vi "OP600ZP_CLUSTER_ISO.vi"(5 "Tableau 3":string[][](array[string]), 10 "Numérique en entrée":i32, 11 "MESURES ISO":cluster{string, string, string, string}) -> (1 "Chaîne":string, 2 "Tableau 2":string[][](array[string]), 3 "Numérique en sortie":i32, 4 "Tableau":bool[](array[boolean]))   [LabVIEW 2020]
uses:
  VG/PackType.vi
  OP500/SubVI/OP500ZP_VGConf.vi
  OP600ZP_VGConf.vi
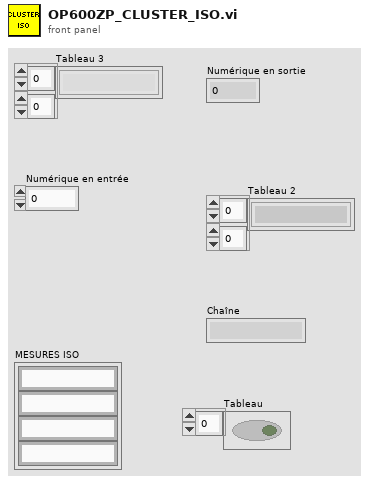
[diagram p1: front panel]
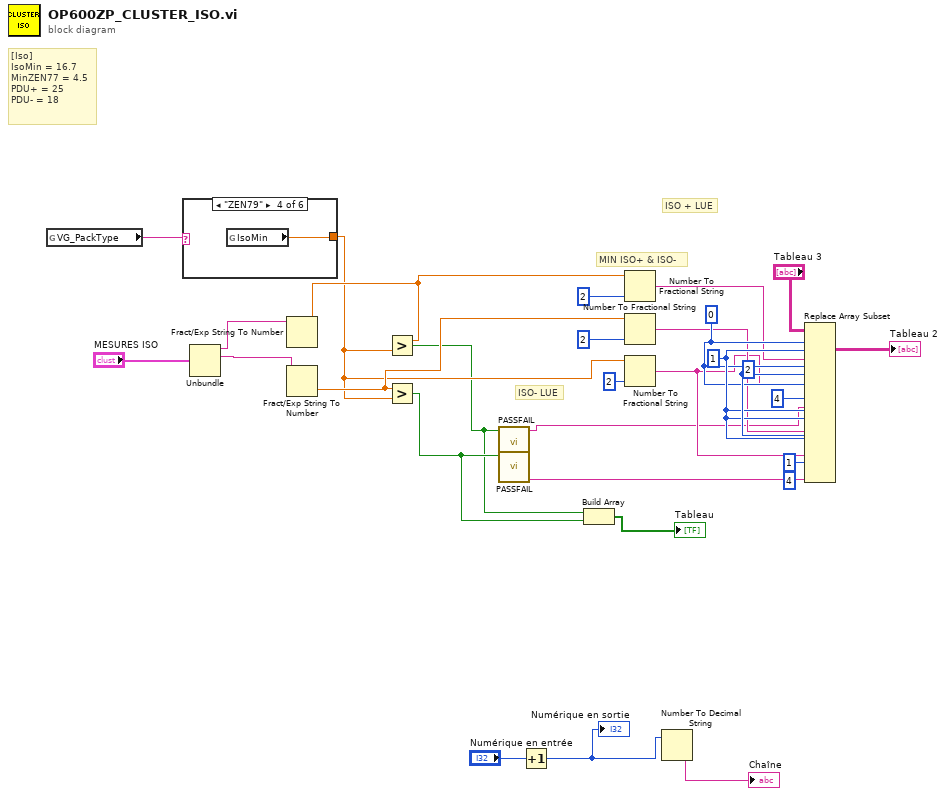
[diagram p0: block diagram]
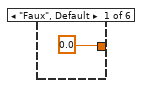
[diagram p2: hidden frame]
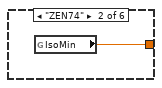
[diagram p3: hidden frame]
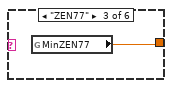
[diagram p4: hidden frame]
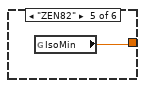
[diagram p5: hidden frame]
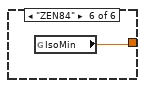
[diagram p6: hidden frame]
diagram:
  w29 = 2 ("disabled index (col)")
  w28 = 1 ("disabled index (col)")
  w26 = 0 ("index (row)")
  # "[Iso]\nIsoMin = 16.7\nMinZEN77 = 4.5\nPDU+ = 25\nPDU- = 18"
  # "ISO- LUE"
  # "ISO + LUE"
  # "MIN ISO+ & ISO-"
  n1 = global read "PackType.vi" "VG_PackType"() -> (w17:string)
  n2 = case shown="\"ZEN79\"" w17 {
    tunnel: [0.0 ("IsoMin") w31 w32 w33 w34 w35] -> w10
    frame "Faux", Default {
    }
    frame "ZEN74" {
      n3 = global read "OP500ZP_VGConf.vi" "IsoMin"() -> (w31:dbl)
    }
    frame "ZEN77" {
      n4 = global read "OP600ZP_VGConf.vi" "MinZEN77"() -> (w32:dbl)
    }
    frame "ZEN79" {
      n5 = global read "OP600ZP_VGConf.vi" "IsoMin"() -> (w33:dbl)
    }
    frame "ZEN82" {
      n6 = global read "OP500ZP_VGConf.vi" "IsoMin"() -> (w34:dbl)
    }
    frame "ZEN84" {
      n7 = global read "OP500ZP_VGConf.vi" "IsoMin"() -> (w35:dbl)
    }
  }
  n8 = Unbundle("MESURES ISO") -> (w19:string, w18:string)  [unwired: 2 out]
  n9 = Fract/Exp String To Number(string=w19) -> (number=w16:dbl)  [unwired: 3 in, 1 out]
  n10 = Fract/Exp String To Number(string=w18) -> (number=w14:dbl)  [unwired: 3 in, 1 out]
  n11 = Greater?(x=w16, y=w10) -> (0:w6:bool)
  n12 = Greater?(x=w14, y=w10) -> (0:w7:bool)
  n13 = call <vilib>:"PASSFAIL.vi"("E"=w6) -> ("S"=w4:string)  [unwired: 10 in]
  n14 = call <vilib>:"PASSFAIL.vi"("E"=w7) -> ("S"=w3:string)  [unwired: 10 in]
  n15 = Increment(x="Numérique en entrée") -> (x+1=w27:i32)
  "Numérique en sortie" <- w27
  n16 = Build Array(w6, w7) -> (→"Tableau":bool[])
  n17 = Number To Fractional String(number=w16, precision (6)=i16 2) -> (F-format string=w12:string)  [unwired: 2 in]
  n18 = Number To Fractional String(number=w14, precision (6)=i16 2) -> (F-format string=w13:string)  [unwired: 2 in]
  n19 = Number To Fractional String(number=w10, precision (6)=i16 2 ("précision (6)")) -> (F-format string=w9:string)  [unwired: 2 in]
  n20 = Number To Decimal String(number=w27) -> (decimal integer string=→"Chaîne":string)  [unwired: 1 in]
  n21 = Replace Array Subset(array="Tableau 3", new element #1=w12, index (row) #1=w26, index (col) #1=w28, new element #2=w9, index (row) #2=w26, index (col) #2=w29, new element #3=w4, index (row) #3=w26, index (col) #3=4 ("indice désactivé (col)"), new element #4=w13, index (row) #4=w28, index (col) #4=w28, new element #5=w9, index (row) #5=w28, index (col) #5=w29, new element #6=w3, index (row) #6=1 ("indice (ligne)"), index (col) #6=4 ("indice désactivé (col)")) -> (→"Tableau 2":string[][])
